vi "Initialize Channel Browser.vi"(6 "Use Channel?":bool, 7 "DisplayFilter":u8(ring)=7 items=["K_CHAN_R", "K_CHAN_W", "K_CHAN_RW", "K_CHAN_VOLT", "K_CHAN_FAULT", "K_ALL", "K_CUSTOM", "K_CHAN_R_VIS", "K_CHAN_W_VIS", "K_CHAN_RW_VIS", "K_CHAN_VOLT_VIS", "K_CHAN_FAULT_VIS"], 8 "error in (no error)":errorcluster, 9 "NodeName":string, 10 "Browser Ref":refnum<k24>, 11 "Item Ref in":T2 format="%.0x") -> (0 "error out":errorcluster, 2 "Browser Ref":T1, 3 "Item Ref out":T2 format="%.0x")   [LabVIEW 2019, in "Control Addon System Explorer.lvlib"]
uses:
  Control Addon System Explorer.lvlib
  <vilib>/NI VeriStand/Custom Device API/Custom Device Item Ref.ctl
  NationalInstruments.VeriStand.SystemStorageUI
  <vilib>/NI VeriStand/UI Controls/Single Node Browser/Single Node Browser Ref.ctl
  NationalInstruments.VeriStand.SystemStorage
  <vilib>/NI VeriStand/Custom Device API/Get Item Property (Dependent Node Pointer).vi
  <vilib>/NI VeriStand/Custom Device Tools/Custom Device Utility Library/Custom Device Utility Library.lvlib
  <vilib>/NI VeriStand/Custom Device API/Custom Device API.lvlib
  <vilib>/NI VeriStand/UI Controls/Single Node Browser/NI_VS UI Single Node Browser.lvlib
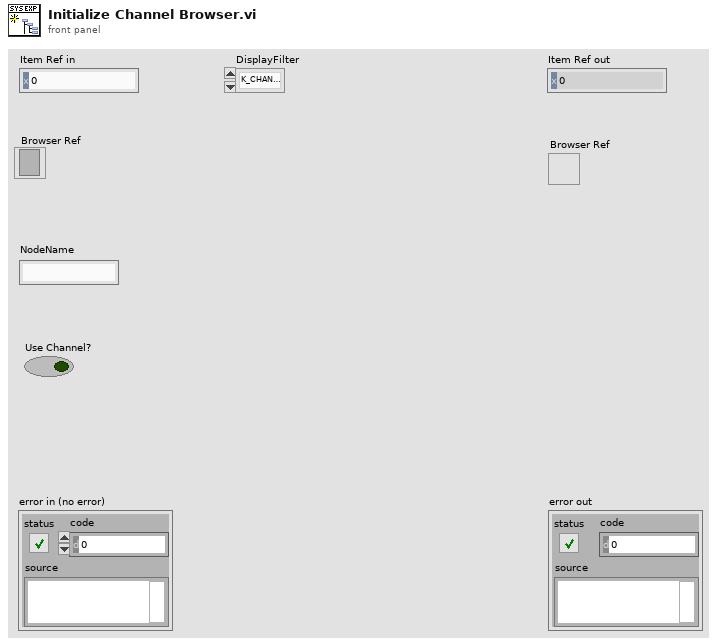
[diagram p1: front panel]
types:
  T1 = typedef "NI_VS UI Single Node Browser.lvlib/Single Node Browser Ref.ctl" = refnum<k24>
  T2 = typedef "Custom Device API.lvlib/Custom Device Item Ref.ctl" = u64
  T3 = typedef "Custom Device API.lvlib/Custom Device Pointer.ctl" = refnum<k24>
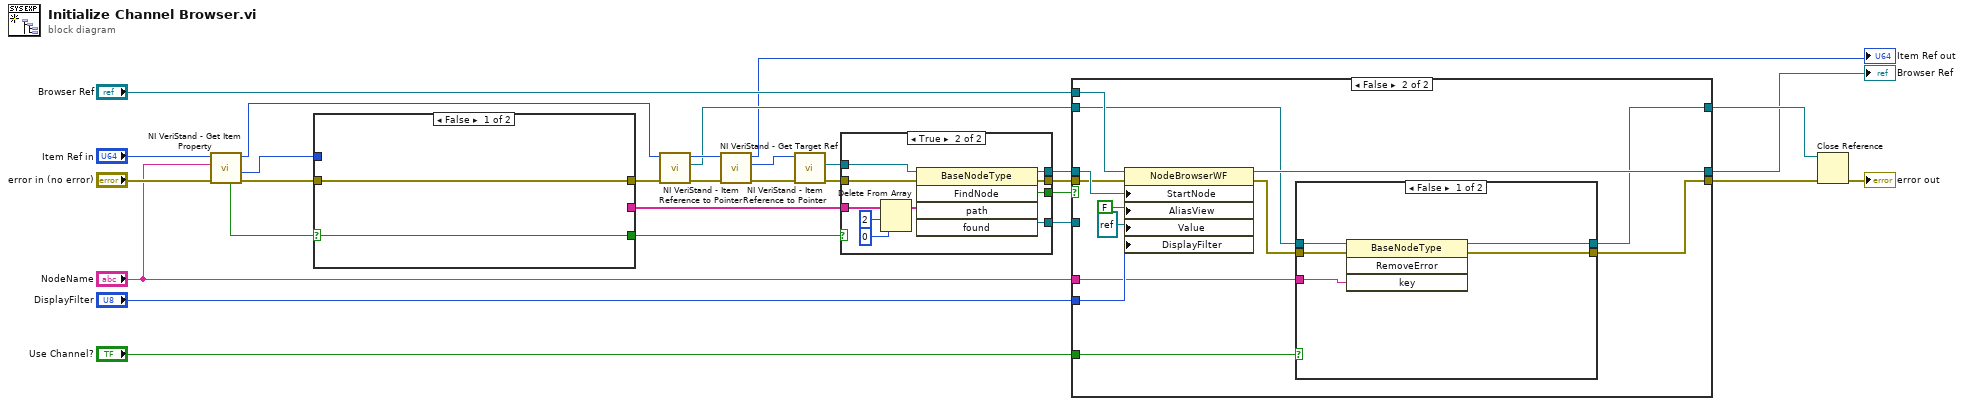
[diagram p0: block diagram]
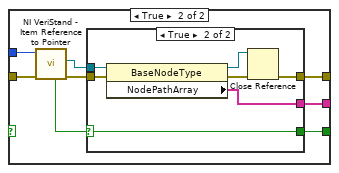
[diagram p2: hidden frame]
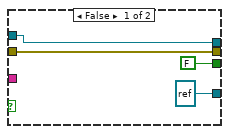
[diagram p4: hidden frame]
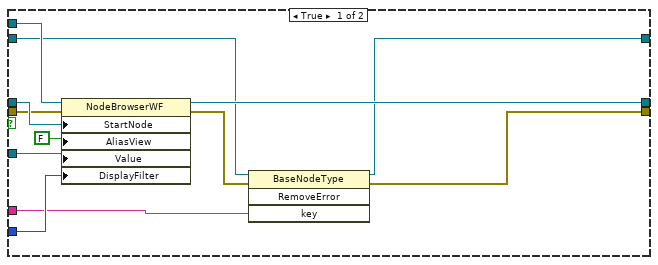
[diagram p5: hidden frame]
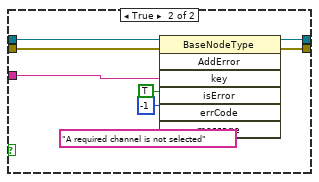
[diagram p6: hidden frame]
diagram:
  n1 = call-poly <vilib>:"NI VeriStand - Get Item Property.vi"("error in (no error)"="error in (no error)", "Property Name"="NodeName", "Item Ref in"="Item Ref in") -> ("error out"=w7:errorcluster, "Dependent Node Ref"=w8:T2, "Item Ref out"=w12:T2, "Found"=w4:bool)  [unwired: 5 in]
  n2 = case shown="False" w4 {
    selector: w4 -> [w30 _]
    tunnel: w8 -> [_ w39]
    tunnel: w7 -> [w31 w38]
    tunnel: [w31 w35] -> w6
    tunnel: [_ w34] -> w3
    tunnel: [w30 w32] -> w5
    frame False {
    }
    frame True {
      n3 = call <vilib>:"NI VeriStand - Item Reference to Pointer.vi"("error in (no error)"=w38, "Item Ref in"=w39) -> ("error out"=w36:errorcluster, "Node Pointer"=w37:T3, "Found"=w33:bool)  [unwired: 6 in, 1 out]
      n4 = case shown="True" w33 {
        selector: w33 -> [w41 w45]
        tunnel: w37 -> [_ w48]
        tunnel: w36 -> [w40 w47]
        tunnel: [w40 w43] -> w35
        tunnel: [_ w46] -> w34
        tunnel: [w41 w45] -> w32
        frame False {
        }
        frame True {
          n5 = property class="BaseNodeType"(reference=w48, error in=w47) -> (reference out=w42:T3, error out=w44:errorcluster, "NodePathArray"=w46:string[])
          n6 = Close Reference(reference=w42, error in (no error)=w44) -> (error out=w43:errorcluster)
        }
      }
    }
  }
  n7 = call <vilib>:"NI VeriStand - Item Reference to Pointer.vi"("error in (no error)"=w6, "Item Ref in"=w12) -> ("error out"=w19:errorcluster, "Node Pointer"=w16:T3, "Item Ref out"=w17:T2)  [unwired: 6 in, 1 out]
  n8 = call <vilib>:"NI VeriStand - Get Target Ref.vi"("error in"=w19, "Item Ref in"=w17) -> ("error out"=w29:errorcluster, "Target Ref"=w22:T2, "Item Ref out"=→"Item Ref out":T2)  [unwired: 6 in, 1 out]
  n9 = call <vilib>:"NI VeriStand - Item Reference to Pointer.vi"("error in (no error)"=w29, "Item Ref in"=w22) -> ("error out"=w24:errorcluster, "Node Pointer"=w23:T3)  [unwired: 6 in, 2 out]
  n10 = case shown="True" w5 {
    tunnel: [refnum<k24> refnum ("Value") w62] -> w27
    tunnel: [w51 w61] -> w26
    tunnel: [w52 w60] -> w25
    tunnel: w24 -> [w52 w57]
    tunnel: w23 -> [w51 w59]
    tunnel: [FALSE ("FindNode") w58] -> w21
    tunnel: w3 -> [_ w54]
    frame False {
    }
    frame True {
      n11 = Delete From Array(array=w54, length=2, index=0) -> (array with subset deleted=w53:string[])  [unwired: 1 out]
      n12 = invoke class="BaseNodeType" method="FindNode"(reference=w59, error in=w57, "path"=w53) -> (reference out=w61:T3, error out=w60:errorcluster, "FindNode"=w58:bool, "found"=w62:refnum<k24>)  [unwired: 2 in, 1 out]
    }
  }
  n13 = case shown="False" w21 {
    tunnel: "DisplayFilter" -> [w70 w82]
    tunnel: "Browser Ref" -> [w74 w87]
    tunnel: [w66 w79] -> w2
    tunnel: w26 -> [w73 w86]
    tunnel: w25 -> [w72 w85]
    tunnel: w27 -> [w71 _]
    tunnel: [w68 w84] -> w1
    tunnel: "Use Channel?" -> [_ w78]
    tunnel: w16 -> [w65 w77]
    tunnel: [w64 w76] -> w14
    tunnel: "NodeName" -> [w63 w75]
    frame True {
      n14 = property class="NodeBrowserWF"(reference=w74, error in=w72, "StartNode"=w73, "AliasView"=FALSE, "Value"=w71, "DisplayFilter"=w70) -> (reference out=w68:refnum<k24>, error out=w67:errorcluster)
      n15 = invoke class="BaseNodeType" method="RemoveError"(reference=w65, error in=w67, "key"=w63) -> (reference out=w64:T3, error out=w66:errorcluster)  [unwired: 1 in, 2 out]
    }
    frame False {
      n16 = property class="NodeBrowserWF"(reference=w87, error in=w85, "StartNode"=w86, "AliasView"=FALSE, "Value"=refnum<k24> refnum, "DisplayFilter"=w82) -> (reference out=w84:refnum<k24>, error out=w80:errorcluster)
      n17 = case shown="False" w78 {
        tunnel: w80 -> [w92 w96]
        tunnel: [w91 w100] -> w79
        tunnel: w77 -> [w90 w97]
        tunnel: [w89 w94] -> w76
        tunnel: w75 -> [w88 w93]
        frame False {
          n18 = invoke class="BaseNodeType" method="RemoveError"(reference=w90, error in=w92, "key"=w88) -> (reference out=w89:T3, error out=w91:errorcluster)  [unwired: 1 in, 2 out]
        }
        frame True {
          n19 = invoke class="BaseNodeType" method="AddError"(reference=w97, error in=w96, "key"=w93, "isError"=TRUE, "errCode"=-1, "message"="A required channel is not selected") -> (reference out=w94:T3, error out=w100:errorcluster)  [unwired: 1 in, 5 out]
        }
      }
    }
  }
  "Browser Ref" <- w1
  n20 = Close Reference(reference=w14, error in (no error)=w2) -> (error out=→"error out":errorcluster)
